vi "AMX-读取电源线头正反面产品参数信息.vi"(8 "错误输入（无错误）":errorcluster, 11 "LoadProductName":string) -> (0 "错误输出":errorcluster)   [LabVIEW 2017]
uses:
  Global System.vi
  <vilib>/Utility/xml.llb/Read From XML File(string).vi
panel:
  out "连接的字符串":string
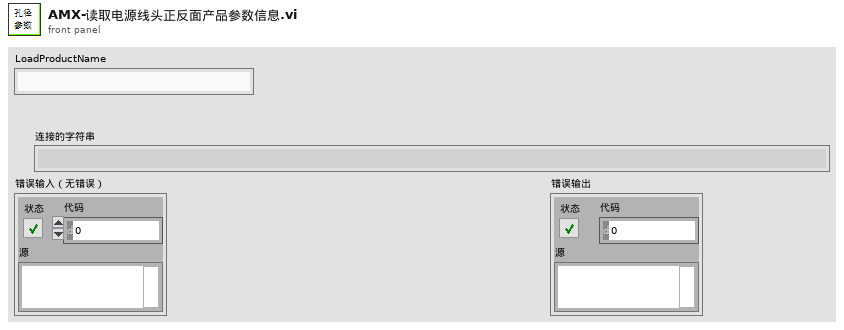
[diagram p1: front panel]
types:
  T1 = typedef "Edge Options.ctl" = cluster{"Edge Polarity":T2, "Kernel Size":u32, "Width":u32, "Minimum Edge Strength":sgl, "Interpolation Type":enum32{"Zero Order", "Bilinear", "Quadratic", "Cubic", "Bilinear Fixed"}, "Data Processing Method":enum32{"Average", "Median"}}
  T2 = typedef "Edge Polarity.ctl" = u32
  T3 = typedef "IMAQ Circle" = cluster{"Center X":i32, "Center Y":i32, "Inner Radius":i32, "Outer Radius":i32, "Start Angle":dbl, "End Angle":dbl}
  T4 = cluster{"圆参数1":cluster{"Search  Direction":u32, "Edge Options":T1, "Show Search Area":bool, "Show Search Lines":bool, "Show Edges Found":bool, "Show Result":bool, "Search Area Color":u32, "Search Lines Color":u32, "Edge Locations Color":u32, "Result Color":u32, "Overlay Group Name":string}, "圆参数":cluster{"Process":enum16{"Get First Edge", "Get First + Last Edge", "Get All Edges", "Get Best Edge"}, "Step Size":i32, "Max Pixel Radius":i32}, "圆环ROI设定":T3, "Show Search Area":bool, "Show Search Lines":bool, "Show Edges Found":bool, "Show Result":bool, "200次模板表格":path, "GRR模板表格":path, "孔径规格":cluster{"孔径上限":string, "孔径标准值":string, "孔径下限":string}}
  T5 = cluster{"IsNorImage":bool, "Exposure Values":u32, "ImagePath":path}
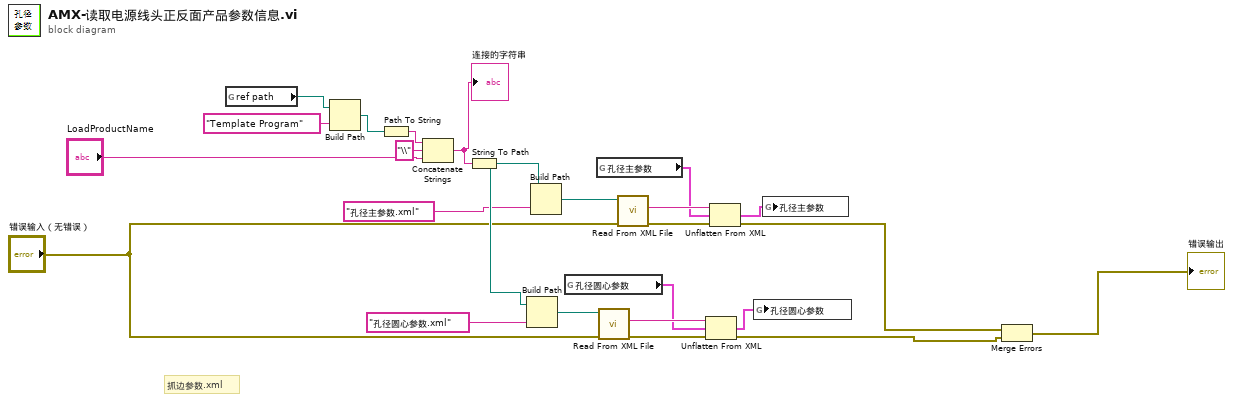
[diagram p0: block diagram]
diagram:
  # "抓边参数.xml"
  n1 = global read "Global System.vi" "ref path"() -> (w23:path)
  n2 = Build Path(base path=w23, name or relative path="Template Program" ("名称或相对路径")) -> (appended path=w21:path)
  n3 = Path To String(path=w21) -> (string=w20:string)
  n4 = Concatenate Strings(w20, "\\" ("字符串"), "LoadProductName") -> (w17:string)
  "连接的字符串" <- w17
  n5 = String To Path(string=w17) -> (path=w15:path)
  n6 = Build Path(base path=w15, name or relative path="孔径圆心参数.xml" ("名称或相对路径")) -> (appended path=w10:path)
  n7 = Build Path(base path=w15, name or relative path="孔径主参数.xml" ("名称或相对路径")) -> (appended path=w13:path)
  n8 = global read "Global System.vi" "孔径圆心参数"() -> (w5:T4)
  n9 = global read "Global System.vi" "孔径主参数"() -> (w7:T5)
  n10 = call-poly <vilib>:"Read From XML File.vi"("error in (no error)"="错误输入（无错误）", "XML File Path"=w10) -> ("error out"=w4:errorcluster, "XML Elements"=w11:string)  [unwired: 7 in, 1 out]
  n11 = call-poly <vilib>:"Read From XML File.vi"("XML File Path"=w13) -> ("XML Elements"=w12:string)  [unwired: 8 in, 2 out]
  n12 = Unflatten From XML(xml string=w11, type=w5, error in (no error)=w4) -> (value=w3:T4, error out=w8:errorcluster)
  n13 = Unflatten From XML(xml string=w12, type=w7, error in (no error)="错误输入（无错误）") -> (value=w6:T5, error out=w9:errorcluster)
  n14 = global write "Global System.vi" "孔径圆心参数"(w3) -> ()
  n15 = global write "Global System.vi" "孔径主参数"(w6) -> ()
  n16 = Merge Errors(w9, w8) -> (→"错误输出":errorcluster)
